vi "LAListen.vi"(8 "Error In":errorcluster, 11 "LiteAgent In":T1) -> (0 "Error Out":errorcluster, 1 "Type":string, 2 "EventJson":string, 3 "LiteAgent Out":T1)   [LabVIEW 2017, in "LiteAgentSDK.lvlib"]
uses:
  LiteAgentSDK.lvlib
  C:/Users/Jan/Projects/LiteAgentSDK-LabVIEW/Source/Bin/LiteAgentSDK.LabVIEW.dll
  Bin/LiteAgentSDK.LabVIEW.dll
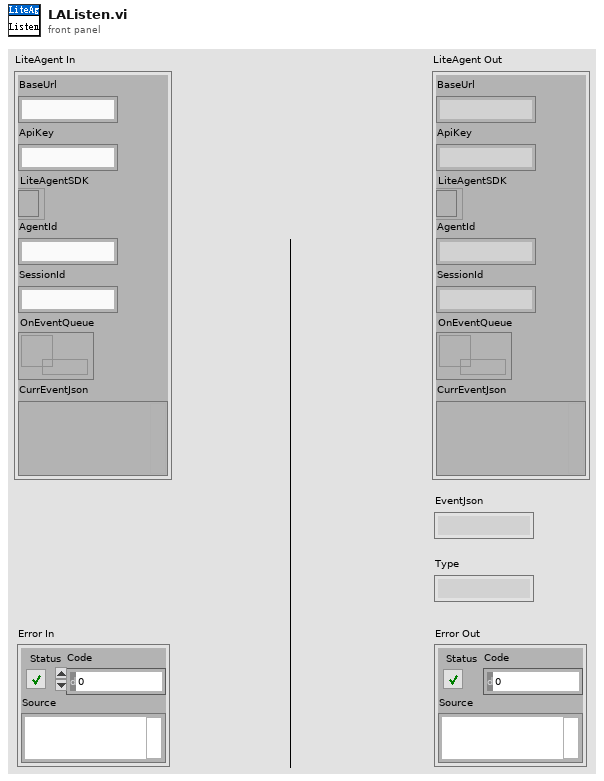
[diagram p1: front panel]
types:
  T1 = cluster{"BaseUrl":string, "ApiKey":string, "LiteAgentSDK":refnum<k24>, "AgentId":string, "SessionId":string, "OnEventQueue":refnum<queue>, "CurrEventJson":variant}
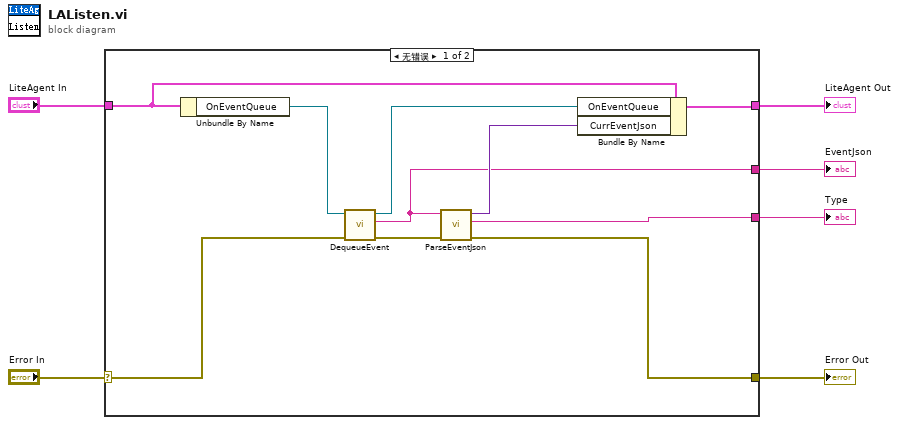
[diagram p0: block diagram]
diagram:
  n1 = case shown="无错误" "Error In" {
    selector: "Error In" -> [w16 w18]
    tunnel: [w8 w18] -> w5
    tunnel: "LiteAgent In" -> [w14 w17]
    tunnel: [w12 w17] -> w3
    tunnel: [w11 _] -> w2
    tunnel: [w7 _] -> w1
    frame No Error {
      n2 = Unbundle By Name(w14) -> ("OnEventQueue"=w15:refnum<queue>)
      n3 = call "DequeueEvent.vi"("Error Input"=w16, "Queue In"=w15) -> ("Error Output"=w10:errorcluster, "EventJson"=w7:string, "Queue Out"=w13:refnum<queue>)  [unwired: 7 in]
      n4 = call "ParseEventJson.vi"("Error In"=w10, "EventJson"=w7) -> ("Error Out"=w8:errorcluster, "Type"=w11:string, "JSON Tree Out"=w9:variant)  [unwired: 7 in]
      n5 = Bundle By Name(cluster=w14, "OnEventQueue"=w13, "CurrEventJson"=w9) -> (w12:T1)
    }
    frame Error {
    }
  }
  "Error Out" <- w5
  "LiteAgent Out" <- w3
  "Type" <- w2
  "EventJson" <- w1
